vi "User Library.vi"(1 "Relative path (.)":path=path "") -> (0 "User Library (+ Relative)":path)   [LabVIEW 2011, in "Path Function.lvlib"]
doc: "Returns the User Library path + relative path."
uses:
  Path Function.lvlib
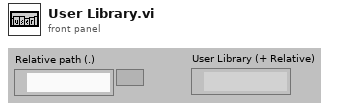
[diagram p1: front panel]
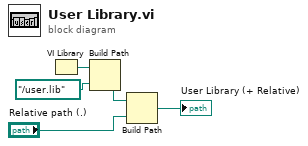
[diagram p0: block diagram]
diagram:
  n1 = VI Library() -> (path=w2:path)
  n2 = Build Path(base path=w2, name or relative path=path "../user.lib" ("Relative path (.)")) -> (appended path=w1:path)
  n3 = Build Path(base path=w1, name or relative path="Relative path (.)") -> (appended path=→"User Library (+ Relative)":path)
